vi "Test shm get Event auth List LV.vi"(8 "error in (no error)":errorcluster, 11 "logevent_authList_Ctl":T1) -> (0 "error out":errorcluster, 2 "function return":i32, 3 "logevent_authList_Ctl out":T1)   [LabVIEW 2018, in "SALLV_Test.lvlib"]
doc: "int Test_shm_getEvent_authListLV(Test_logevent_authListLV *logevent_authList_Ctl );"
uses:
  SALLV_Test.lvlib
  SALLV_Test.so
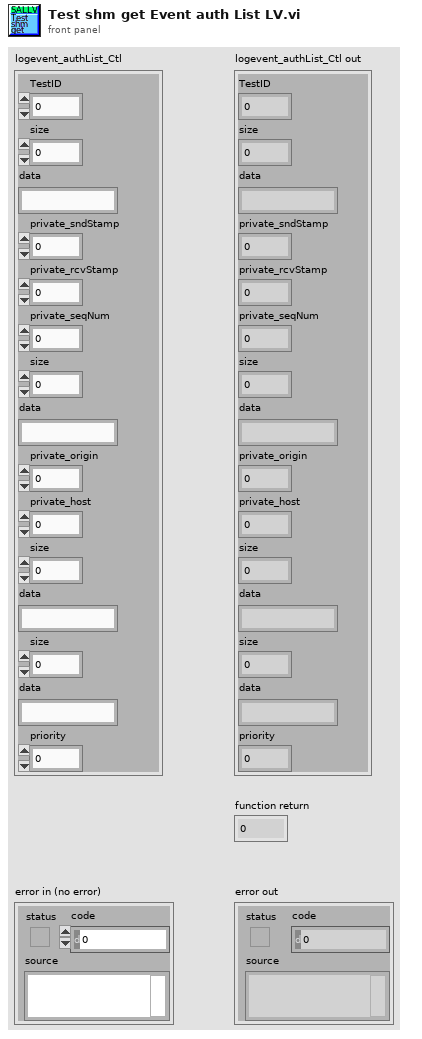
[diagram p1: front panel]
types:
  T1 = cluster{"TestID":i32, "size":i32, "data":string, "private_sndStamp":dbl, "private_rcvStamp":dbl, "private_seqNum":i32, "size":i32, "data":string, "private_origin":i32, "private_host":i32, "size":i32, "data":string, "size":i32, "data":string, "priority":i32}
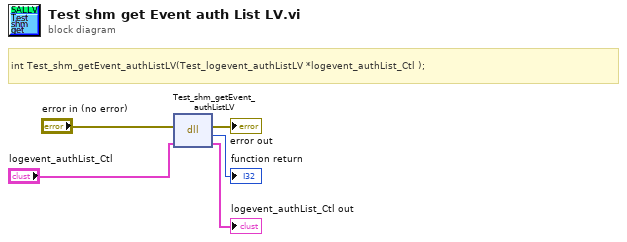
[diagram p0: block diagram]
diagram:
  # "int Test_shm_getEvent_authListLV(Test_logevent_authListLV *logevent_authList_Ctl );"
  n1 = dll-call lib="home/ttsai/Documents/salTestLabViewApi/SALLV_Test/SALLV_Test.*" fn="Test_shm_getEvent_authListLV"(error in="error in (no error)", "logevent_authList_Ctl"="logevent_authList_Ctl") -> (error out=→"error out":errorcluster, →"function return":i32, "logevent_authList_Ctl"=→"logevent_authList_Ctl out":T1)  [unwired: 2 in, 1 out]
